vi "Update BlockNode State.vi"(8 "error in (no error)":errorcluster, 11 "State in":T1 {"BlockNodeState"."Draw Style" items=["FunctionBlock", "ExpressVI", "Variable", "Elemental I/O", "32x32 Icon", "FunctionBlockCompact"]; "BlockNodeState"."Terminal Data"."Terminal Flags" format="%.0b"}) -> (0 "error out":errorcluster, 3 "State out":T1 {"BlockNodeState"."Draw Style" items=["FunctionBlock", "ExpressVI", "Variable", "Elemental I/O", "32x32 Icon", "FunctionBlockCompact"]; "BlockNodeState"."Terminal Data"."Terminal Flags" format="%.0b"})   [LabVIEW 2017, in "NI_Robotics_Create Steering Frame.xnode"]
uses:
  <vilib>/robotics/Steering/Create Steering Frame/NI_Robotics_Create Steering Frame.xnode
  <vilib>/robotics/Steering/Create Steering Frame/State.ctl
  <vilib>/BlockNodeSupport/BlockNodeState.ctl
  <vilib>/BlockNodeSupport/TerminalData.ctl
  <vilib>/picture/picture.llb/imagedata.ctl
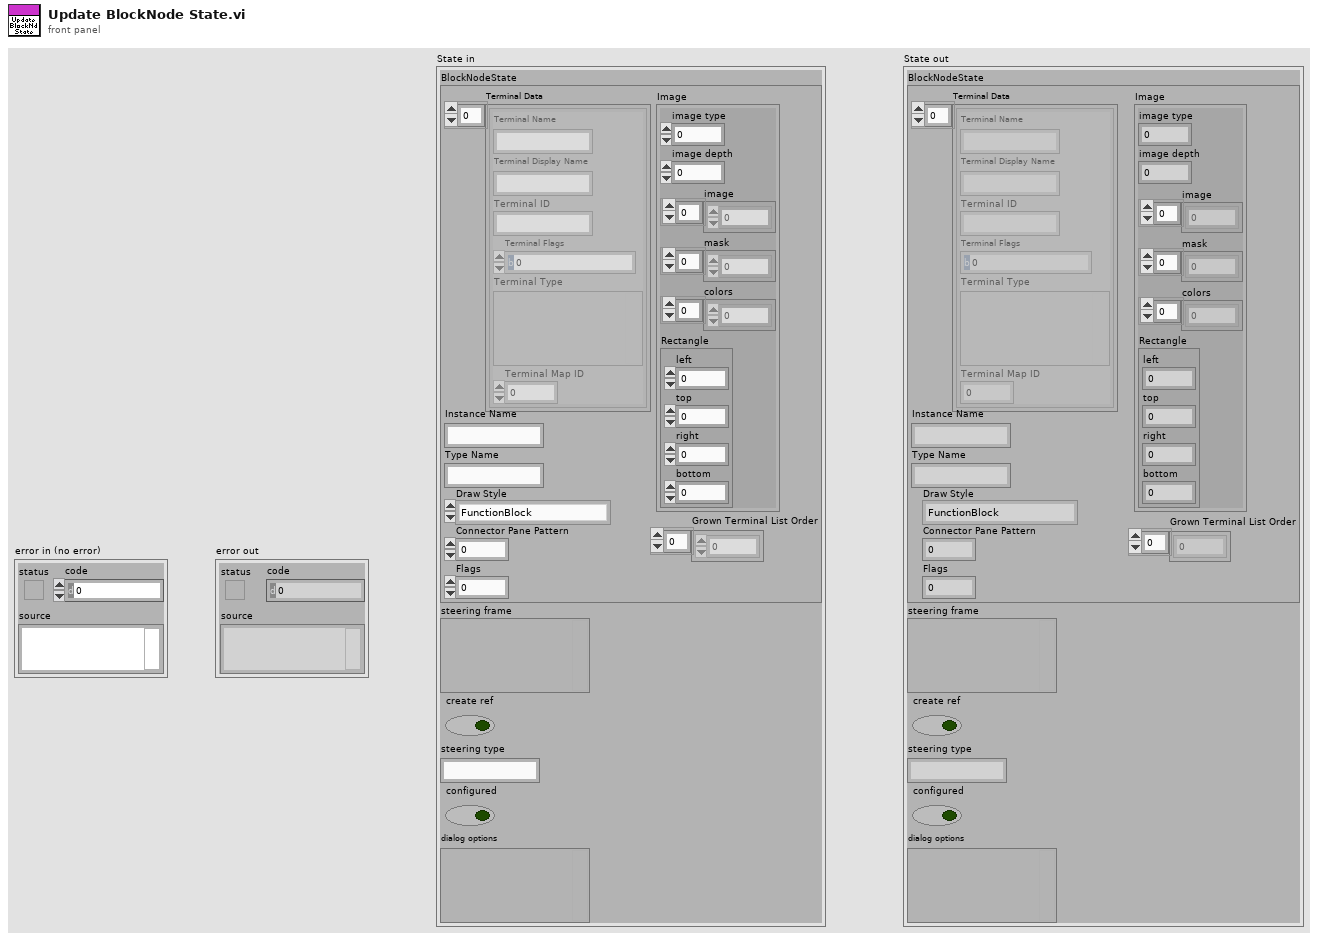
[diagram p1: front panel]
types:
  T1 = typedef "NI_Robotics_Create Steering Frame.xnode/State.ctl" = cluster{"BlockNodeState":T2, "steering frame":variant, "create ref":bool, "steering type":string, "configured":bool, "dialog options":variant}
  T2 = typedef "BlockNodeState.ctl" = cluster{"Terminal Data":T3[], "Instance Name":string, "Type Name":string, "Draw Style":i32, "Connector Pane Pattern":i32, "Flags":i32, "Grown Terminal List Order":i32[], "Image":T4}
  T3 = typedef "TerminalData.ctl" = cluster{"Terminal Name":string, "Terminal Display Name":string, "Terminal ID":string, "Terminal Flags":i32, "Terminal Type":variant, "Terminal Map ID":i32}
  T4 = typedef "imagedata.ctl" = cluster{"image type":i32, "image depth":i32, "image":u8[], "mask":u8[], "colors":u32[], "Rectangle":cluster{"left":i16, "top":i16, "right":i16, "bottom":i16}}
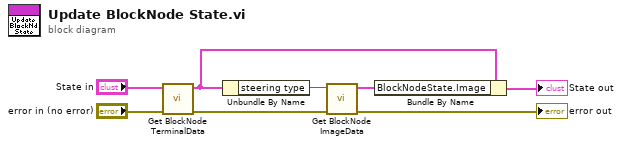
[diagram p0: block diagram]
diagram:
  n1 = call <vilib>:"Get BlockNode TerminalData.vi"("error in (no error)"="error in (no error)", "State in"="State in") -> ("error out"=w5:errorcluster, "State out"=w1:T1)  [unwired: 8 in]
  n2 = Unbundle By Name(w1) -> ("steering type"=w8:string)
  n3 = call <vilib>:"Get BlockNode ImageData.vi"("error in (no error)"=w5, "steering type (\"\")"=w8) -> ("error out"=→"error out":errorcluster, "image data"=w6:T4)  [unwired: 8 in]
  n4 = Bundle By Name(cluster=w1, "BlockNodeState.Image"=w6) -> (→"State out":T1)
